vi "Actor.vi"(11 "Class":refnum<class "DAQmx - Analog Output Multi Sample.lvclass">) -> ()   [LabVIEW 2021, in "DAQmx - Analog Output Multi Sample.lvclass"]
uses:
  DAQmx - Analog Output Multi Sample.lvclass
  C:/TSA/DAQmx-Bus/Source/DAQmx-Bus.lvclass
  DAQmx-Bus.lvclass/DAQmx-Bus.ctl
  DAQmx - Analog Output Multi Sample.lvclass/DAQmx - Analog Output Multi Sample.ctl
  <vilib>/Platform/TimedLoop/XDataNode/timing_clust.ctl
  <vilib>/Platform/TimedLoop/XDataNode/nitl_modes.ctl
  <vilib>/Platform/TimedLoop/XDataNode/wakeup.ctl
  <vilib>/DAQmx/write.llb/DAQmx Write (Analog 1D Wfm NChan NSamp).vi
  Properties/Read DAQmx Task.vi
  Properties/Read Update Rate.vi
  Properties/Read timeout.vi
  Properties/Read Values DVR.vi
  Properties/Read Stop.vi
  Properties/Read Sync.vi
  <vilib>/DAQmx/miscellaneous.llb/DAQmx Fill In Error Info.vi
  <vilib>/platform/TimedLoop/XDataNode/XDataNode.xnode
  <resource>/objmgr/daqmx.rc
  <vilib>/Platform/TimedLoop/XDataNode/XDNodeRunTimeDep.lvlib
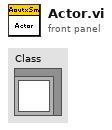
[diagram p1: front panel]
types:
  T1 = typedef "XDNodeRunTimeDep.lvlib/timing_clust.ctl" = cluster{"Expected End [f-1]":u64, "Actual End [f-1]":u64, "Finished Late? [f-1]":bool, "Expected End [i-1]":u64, "Actual End [i-1]":u64, "Finished Late? [i-1]":bool, "Expected Start [i]":u64, "Actual Start [i]":u64, "Expected Start [f]":u64, "Actual Start [f]":u64, "Source Name":string, "Structure Name":string, "Period":i64, "Deadline":i64, "Offset":i64, "Start":i64, "Priority":i32, "Timeout":i32, "Mode":T2, "Wakeup Reason":T3, "Error":errorcluster, "Source Type":string, "Secondary Source Type":string, "Global End Time":u64, "Global Start Time":u64, "Frame Duration":u64, "Iteration Duration":u64, "Assigned CPU":i32, "I/O Scan Engine Mode":u32}
  T2 = typedef "XDNodeRunTimeDep.lvlib/nitl_modes.ctl" = enum32{"No Change", "Process missed periods, maintain original phase", "Discard missed periods, maintain original phase", "Process missed periods, ignore original phase", "Discard missed periods, ignore original phase"}
  T3 = typedef "XDNodeRunTimeDep.lvlib/wakeup.ctl" = enum32{"Normal", "Aborted", "Asynchronous wakeup", "Timing source error", "Timed loop error", "Timeout"}
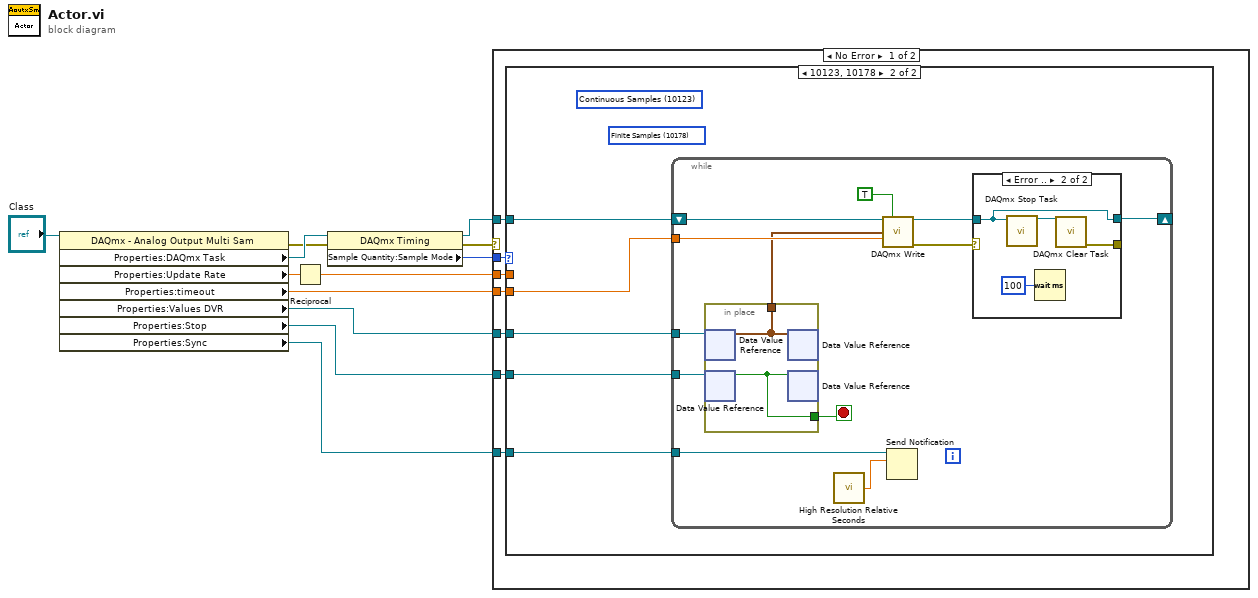
[diagram p0: block diagram]
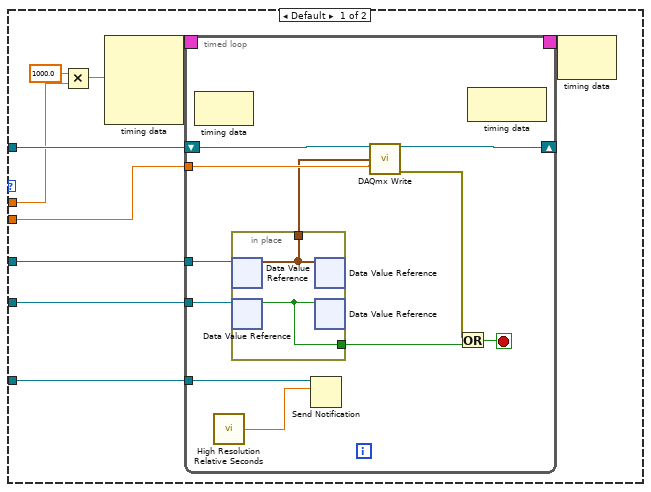
[diagram p2: hidden frame]
diagram:
  n1 = property class="DAQmx - Analog Output Multi Sam"(reference="Class") -> (error out=w7:errorcluster, "Properties:DAQmx Task"=w8:refnum<k21>, "Properties:Update Rate"=w5:dbl, "Properties:timeout"=w11:dbl, "Properties:Values DVR"=w10:refnum<data-value>, "Properties:Stop"=w12:refnum<data-value>, "Properties:Sync"=w9:refnum<notifier>)  [unwired: 1 in, 1 out]
  n2 = Reciprocal(x=w5) -> (1/x=w4:dbl)
  n3 = property class="DAQmx Timing"(reference=w8, error in=w7) -> (reference out=w1:refnum<k21>, error out=w2:errorcluster, "Sample Quantity:Sample Mode"=w6:i32)
  n4 = case shown="No Error" w2 {
    tunnel: w12 -> [w19 _]
    tunnel: w11 -> [w18 _]
    tunnel: w10 -> [w17 _]
    tunnel: w9 -> [w16 _]
    tunnel: w1 -> [w15 _]
    tunnel: w6 -> [w14 _]
    tunnel: w4 -> [w13 _]
    frame No Error {
      n5 = case shown="10123, 10178" w14 {
        tunnel: w19 -> [w29 w53]
        tunnel: w18 -> [w28 w52]
        tunnel: w17 -> [w27 w51]
        tunnel: w16 -> [w26 w50]
        tunnel: w15 -> [w25 w49]
        tunnel: w13 -> [w22 _]
        frame Default {
          n6 = Multiply(x=1000.0, y=w22) -> (x*y=w20:dbl)
          n7 = node-c288(w20) -> (w24:T1)  [unwired: 3 in]
          n8 = timed-loop {
            shift-right: [w35] -> _
            shift-left: w25 -> [w36]
            tunnel: w29 -> [w40]
            tunnel: w28 -> [w34]
            tunnel: w27 -> [w39]
            tunnel: w26 -> [w37]
            timing: w24 -> [_]
            timing-out: [_] -> w23
            stop <- w30 stop-if-true
            n9 = node-c288() -> ()  [unwired: 1 in, 1 out]
            n10 = call <vilib>:"High Resolution Relative Seconds.vi"() -> ("relative seconds"=w38:dbl)
            n11 = in-place {
              in-place-border: [w44] -> w31
              in-place-border: [w43] -> w33
              n12 = in-place-dvr #1(w39) -> (w43:waveform(dbl)[])  [unwired: 1 out]
              n13 = in-place-dvr #2(w40) -> (w44:bool)  [unwired: 1 out]
              n14 = in-place-dvr #1(w43) -> ()  [unwired: 2 out]
              n15 = in-place-dvr #2(w44) -> ()  [unwired: 2 out]
            }
            n16 = Send Notification(notification=w38, notifier=w37) -> ()  [unwired: 1 in, 2 out]
            n17 = call-poly <vilib>:"DAQmx Write.vi"("task/channels in"=w36, "data"=w33, "timeout"=w34) -> ("task out"=w35:refnum<k21>, "error out"=w32:errorcluster)  [unwired: 10 in, 1 out]
            n18 = Or(x=w32, y=w31) -> (x .or. y?=w30:bool)
            n19 = node-c288() -> ()  [unwired: 1 in, 1 out]
          }
          n20 = node-c288(w23) -> ()  [unwired: 1 out]
        }
        frame 10123, 10178 {
          (unwired) 10178 items=["Finite Samples"=10178, "Continuous Samples"=10123, "Hardware Timed Single Point"=12522] ("SampQuant.SampMode")
          (unwired) 10123 items=["Finite Samples"=10178, "Continuous Samples"=10123, "Hardware Timed Single Point"=12522] ("SampQuant.SampMode")
          n21 = while {
            shift-right: [w56] -> _
            shift-left: w49 -> [w54]
            tunnel: w53 -> [w65]
            tunnel: w52 -> [w62]
            tunnel: w51 -> [w64]
            tunnel: w50 -> [w63]
            stop <- w61 stop-if-true
            n22 = in-place {
              in-place-border: [w73] -> w61
              in-place-border: [w72] -> w59
              n23 = in-place-dvr #3(w64) -> (w72:waveform(dbl)[])  [unwired: 1 out]
              n24 = in-place-dvr #4(w65) -> (w73:bool)  [unwired: 1 out]
              n25 = in-place-dvr #3(w72) -> ()  [unwired: 2 out]
              n26 = in-place-dvr #4(w73) -> ()  [unwired: 2 out]
            }
            n27 = call <vilib>:"High Resolution Relative Seconds.vi"() -> ("relative seconds"=w60:dbl)
            n28 = call-poly <vilib>:"DAQmx Write.vi"("task/channels in"=w54, "auto start"=TRUE, "data"=w59, "timeout"=w62) -> ("task out"=w57:refnum<k21>, "error out"=w55:errorcluster)  [unwired: 9 in, 1 out]
            n29 = Send Notification(notification=w60, notifier=w63) -> ()  [unwired: 1 in, 2 out]
            n30 = case shown="Error .." w55 {
              selector: w55 -> [w66 _]
              tunnel: w57 -> [w67 w69]
              tunnel: [w67 w69] -> w56
              tunnel: [w66 w68] -> _
              frame No Error {
              }
              frame Error {
                n31 = call <vilib>:"DAQmx Stop Task.vi"("task/channels in"=w69) -> ("task out"=w70:refnum<k21>)  [unwired: 13 in, 1 out]
                n32 = Wait (ms)(milliseconds to wait=u32 100) -> ()  [unwired: 1 out]
                n33 = call <vilib>:"DAQmx Clear Task.vi"("task in"=w70) -> ("error out"=w68:errorcluster)  [unwired: 14 in]
              }
            }
          }
        }
      }
    }
    frame Error {
    }
  }
